vi "end kml.vi"(6 "KML IN":string, 7 "Path":path) -> ()   [LabVIEW 2015, in "Biblioteka moduł map v3.lvlib" / "KML.lvlib"]
uses:
  KML.lvlib
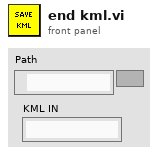
[diagram p1: front panel]
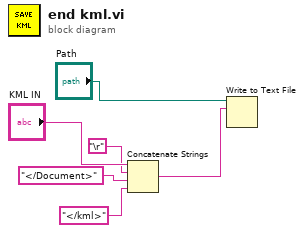
[diagram p0: block diagram]
diagram:
  n1 = Concatenate Strings("KML IN", "\r", "</Document>", "</kml>") -> (w4:string)
  n2 = Write to Text File(file (use dialog)="Path", text=w4) -> ()  [unwired: 2 in, 3 out]
